vi "Scan DQMH Modules from Project.vi"(6 "TreeControl in":refnum<vi>, 7 "Data Cluster In":T2={"Project"=refnum, "Current Selection"={"Library"=refnum, "VI"=refnum}, "Module ID"=-1, "Tree Selection"=""}, 8 "error in":errorcluster, 11 "Scan DQMH Modules Argument":T1) -> (0 "error out":errorcluster, 5 "Data Cluster Out":T2={"Project"=refnum, "Current Selection"={"Library"=refnum, "VI"=refnum}, "Module ID"=-1, "Tree Selection"=""})   [LabVIEW 2020, in "Panther Dashboard.lvlib"]
doc: "Gets the Singleton and Cloneable references and creates a list of each type of DQMH Modules"
uses:
  Panther Dashboard.lvlib
  Module Data--cluster.ctl
  Class/Project/Project.lvclass
  C:/GitClones/PantherDashboard/src/LabVIEW/Panther Dashboard/Class/LabVIEWItem/LabVIEWItem.lvclass
  Class/Library/Library.lvclass
  Class/VI/VI.lvclass
  Scan DQMH Modules Argument--cluster.ctl
  Class/LabVIEWItem/LabVIEWItem.lvclass/LabVIEWItem.ctl
  Class/LabVIEWItem/Read Item Tag.vi
  Class/LabVIEWItem/Read Item Path.vi
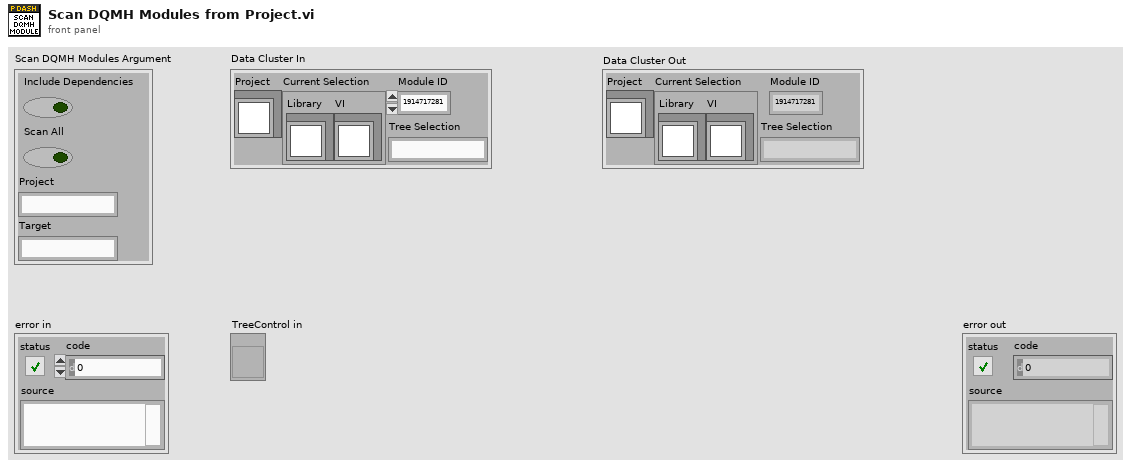
[diagram p1: front panel]
types:
  T1 = typedef "Panther Dashboard.lvlib/Scan DQMH Modules Argument--cluster.ctl" = cluster{"Include Dependencies":bool, "Scan All":bool, "Project":string, "Target":string}
  T2 = typedef "Panther Dashboard.lvlib/Module Data--cluster.ctl" = cluster{"Project":refnum<class "Project.lvclass">, "Current Selection":cluster{"Library":refnum<class "Library.lvclass">, "VI":refnum<class "VI.lvclass">}, "Module ID":i32, "Tree Selection":string}
  T3 = typedef "DQMH_Scripting API.lvlib/Module Information--cluster.ctl" = cluster{"Library":refnum<vi>, "Qualified Name":string, "Path":path, "Cloneable":bool, "Under Dependencies":bool}
  T4 = typedef "Tree Map.lvlib/Tree Map Data.ctl" = map{string, cluster{"Child Paths Set":set{string}, "Name":string, "Data":string, "Attributes":map{string, string}}}
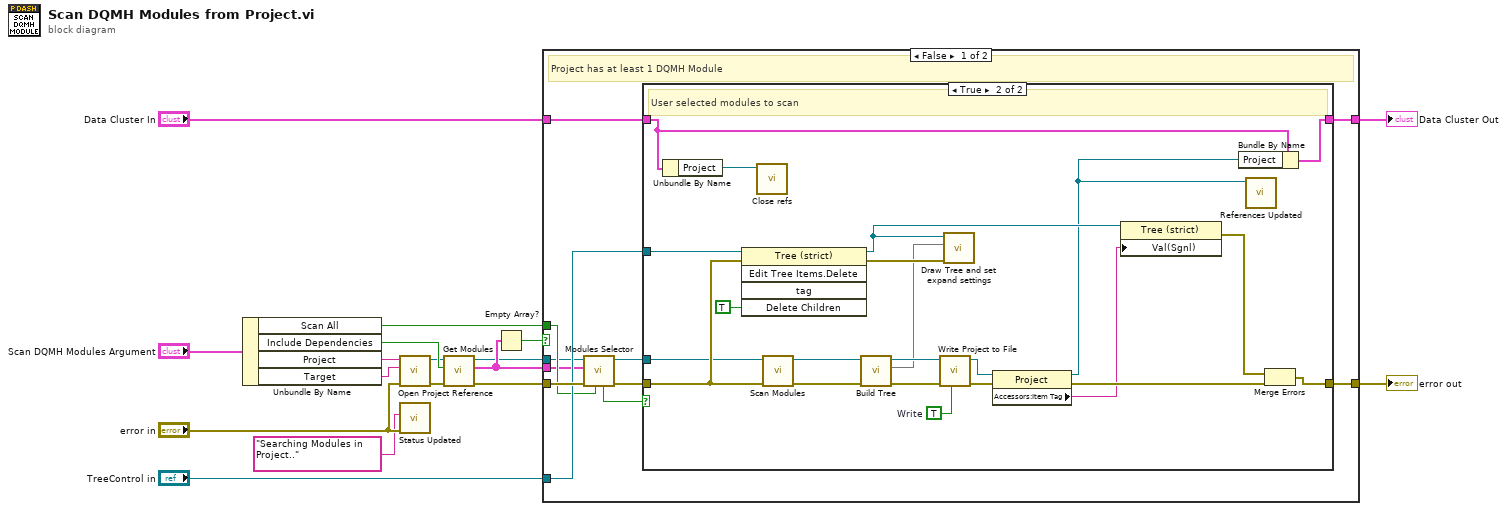
[diagram p0: block diagram]
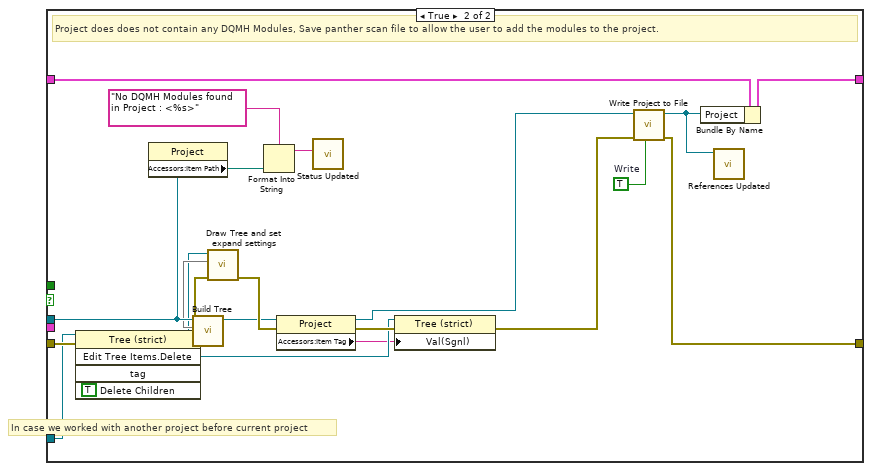
[diagram p3: hidden frame]
diagram:
  n1 = Unbundle By Name("Scan DQMH Modules Argument") -> ("Scan All"=w5:bool, "Include Dependencies"=w6:bool, "Project"=w4:string, "Target"=w3:string)
  n2 = call "Open Project Reference.vi"("error in"="error in", "Target Selection"=w3, "Project Selection"=w4) -> ("error out"=w16:errorcluster, "Project"=w2:refnum<class "Project.lvclass">)  [unwired: 7 in]
  n3 = call "Status Updated.vi"("error in (no error)"="error in", "Status"="Searching Modules in Project..") -> ()  [unwired: 9 in, 1 out]
  n4 = call "Get Modules.vi"("error in"=w16, "Include Dependencies"=w6, "Project in"=w2) -> ("error out"=w15:errorcluster, "DQMH Modules"=w7:T3[], "Project out"=w1:refnum<class "Project.lvclass">)  [unwired: 6 in]
  n5 = Empty Array?(array=w7) -> (empty?=w8:bool)
  n6 = case shown="False" w8 {
    tunnel: w15 -> [w27 w74]
    tunnel: [w28 w69] -> w17
    tunnel: w1 -> [w19 w59]
    tunnel: "Data Cluster In" -> [w25 w67]
    tunnel: [w24 w66] -> w12
    tunnel: "TreeControl in" -> [w22 w62]
    tunnel: w7 -> [w20 _]
    tunnel: w5 -> [w21 _]
    frame False {
      # "Project has at least 1 DQMH Module"
      n7 = call "Modules Selector.vi"("Scan All"=w21, "error in"=w27, "DQMH Modules"=w20, "Project In"=w19) -> ("error out"=w26:errorcluster, "Project Out"=w18:refnum<class "Project.lvclass">, "Scan?"=w23:bool)  [unwired: 5 in]
      n8 = case shown="True" w23 {
        tunnel: w25 -> [w29 w39]
        tunnel: [w29 w44] -> w24
        tunnel: w22 -> [_ w43]
        tunnel: w26 -> [w30 w50]
        tunnel: [w30 w47] -> w28
        tunnel: w18 -> [_ w41]
        frame False {
          # "User Cancel Scan process, do not redraw tree and keep previous selection"
        }
        frame True {
          w35 = TRUE  # Write
          # "User selected modules to scan"
          n9 = Unbundle By Name(w39) -> ("Project"=w40:refnum<class "Project.lvclass">)
          n10 = invoke class="Tree (strict)" method="Edit Tree Items.Delete"(reference=w43, error in=w50, "Delete Children"=TRUE ("Delete Children?")) -> (reference out=w34:refnum<vi>, error out=w49:errorcluster)  [unwired: 2 in, 3 out]
          n11 = call "Close refs.vi"("Project"=w40) -> ()  [unwired: 10 in, 1 out]
          n12 = call "Scan Modules.vi"("error in"=w50, "Project In"=w41) -> ("error out"=w52:errorcluster, "Project Out"=w38:refnum<class "Project.lvclass">)  [unwired: 8 in]
          n13 = call "Build Tree.vi"("error in"=w52, "Project in"=w38) -> ("error out"=w48:errorcluster, "Tree Map Out"=w36:T4, "Project Out"=w37:refnum<class "Project.lvclass">)  [unwired: 7 in]
          n14 = call "Write Project to File.vi"("Write"=w35, "error in"=w48, "Project In"=w37) -> ("error out"=w51:errorcluster, "Project Out"=w33:refnum<class "Project.lvclass">)  [unwired: 6 in, 1 out]
          n15 = call "Draw Tree and set expand settings.vi"("error in"=w49, "Tree Map In"=w36, "TreeControl in"=w34) -> ()  [unwired: 8 in, 1 out]
          n16 = property class="Project"(reference=w33, error in=w51) -> (reference out=w32:refnum<class "Project.lvclass">, error out=w45:errorcluster, "Accessors:Item Tag"=w31:string)
          n17 = property class="Tree (strict)"(reference=w34, "Val(Sgnl)"=w31) -> (error out=w46:errorcluster)  [unwired: 1 in, 1 out]
          n18 = Bundle By Name(cluster=w39, "Project"=w32) -> (w44:T2)
          n19 = call "References Updated.vi"("Project"=w32) -> ()  [unwired: 10 in, 1 out]
          n20 = Merge Errors(w46, w45) -> (w47:errorcluster)
        }
      }
    }
    frame True {
      w61 = TRUE  # Write
      # "In case we worked with another project before current project"
      # "Project does does not contain any DQMH Modules, Save panther scan file to allow the user to add the modules to the project."
      n21 = invoke class="Tree (strict)" method="Edit Tree Items.Delete"(reference=w62, error in=w74, "Delete Children"=TRUE ("Delete Children?")) -> (reference out=w57:refnum<vi>, error out=w73:errorcluster)  [unwired: 2 in, 3 out]
      n22 = property class="Project"(reference=w59) -> ("Accessors:Item Path"=w60:path)  [unwired: 1 in, 2 out]
      n23 = call "Build Tree.vi"("error in"=w73, "Project in"=w59) -> ("error out"=w72:errorcluster, "Tree Map Out"=w58:T4, "Project Out"=w55:refnum<class "Project.lvclass">)  [unwired: 7 in]
      n24 = call "Draw Tree and set expand settings.vi"("error in"=w72, "Tree Map In"=w58, "TreeControl in"=w57) -> ("error out"=w71:errorcluster)  [unwired: 8 in]
      n25 = Format Into String(format string="No DQMH Modules found in Project : <%s>", w60) -> (resulting string=w65:string)  [unwired: 2 in, 1 out]
      n26 = property class="Project"(reference=w55, error in=w71) -> (reference out=w54:refnum<class "Project.lvclass">, error out=w68:errorcluster, "Accessors:Item Tag"=w53:string)
      n27 = call "Status Updated.vi"("Status"=w65) -> ()  [unwired: 10 in, 1 out]
      n28 = property class="Tree (strict)"(reference=w57, error in=w68, "Val(Sgnl)"=w53) -> (error out=w70:errorcluster)  [unwired: 1 out]
      n29 = call "Write Project to File.vi"("Write"=w61, "error in"=w70, "Project In"=w54) -> ("error out"=w69:errorcluster, "Project Out"=w56:refnum<class "Project.lvclass">)  [unwired: 6 in, 1 out]
      n30 = Bundle By Name(cluster=w67, "Project"=w56) -> (w66:T2)
      n31 = call "References Updated.vi"("Project"=w56) -> ()  [unwired: 10 in, 1 out]
    }
  }
  "error out" <- w17
  "Data Cluster Out" <- w12
